vi "Items_set.vi"(8 "error in (no error)":errorcluster, 9 "Channels":string[](array[string]), 10 "Stream Group":i32=1 min=1, 11 "OXY_SCPI Reseource In":refnum<visa-resource-name>) -> (0 "error out":errorcluster, 2 "communication_data":T1, 3 "OXY_SCPI Reseource Out":refnum<visa-resource-name>)   [LabVIEW 2020, in "OXYGEN_Datastream.lvlib"]
uses:
  OXYGEN_Datastream.lvlib
  TypeDefs/Cluster_RawCommData.ctl
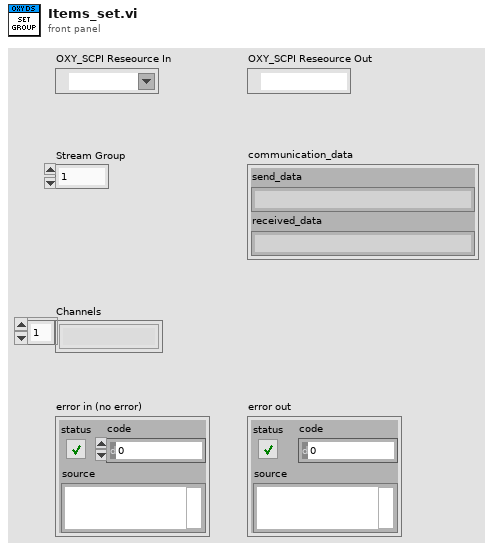
[diagram p1: front panel]
types:
  T1 = typedef "OXYGEN_Datastream.lvlib/Cluster_RawCommData.ctl" = cluster{"send_data":string, "received_data":string}
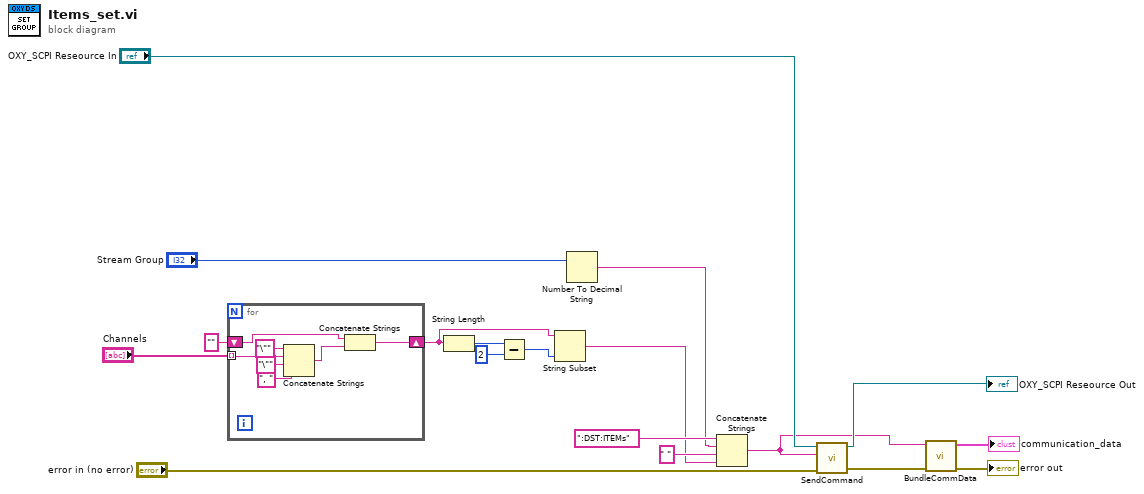
[diagram p0: block diagram]
diagram:
  n1 = for {
    tunnel: "Channels" -> [w25] mode=indexing
    shift-right: [w21] -> w5
    shift-left: "" -> [w19]
    n2 = Concatenate Strings("\"" ("string"), w25, "\"" ("string"), ", " ("string")) -> (w20:string)
    n3 = Concatenate Strings(w19, w20) -> (w21:string)
  }
  n4 = String Length(string=w5) -> (length=w7:i32)
  n5 = Subtract(x=w7, y=2) -> (x-y=w4:i32)
  n6 = String Subset(string=w5, length (rest)=w4) -> (substring=w3:string)  [unwired: 1 in]
  n7 = Number To Decimal String(number="Stream Group") -> (decimal integer string=w10:string)  [unwired: 1 in]
  n8 = Concatenate Strings(":DST:ITEMs", w10, " ", w3) -> (w13:string)
  n9 = call "SendCommand.vi"("error in (no error)"="error in (no error)", "String to Send"=w13, "OXY_SCPI Reseource In"="OXY_SCPI Reseource In") -> ("error out"=w14:errorcluster, "OXY_SCPI Reseource Out"=→"OXY_SCPI Reseource Out":refnum<visa-resource-name>)  [unwired: 7 in]
  n10 = call "BundleCommData.vi"("error in (no error)"=w14, "send_data"=w13) -> ("error out"=→"error out":errorcluster, "communication_data"=→"communication_data":T1)  [unwired: 8 in]
